vi "writeSDOU16.vi"(6 "object sub-index (0)":u8 format="%x", 7 "object index":u16 format="%x", 8 "error in (no error)":errorcluster, 9 "interface object in":refnum<k20>, 10 "inputNumber":u16, 11 "MotorController in":refnum<class "MotorController.lvclass">) -> (0 "error out":errorcluster, 1 "completion code":u32, 2 "interface object out":refnum<k20>, 3 "MotorController out":refnum<class "MotorController.lvclass">)   [LabVIEW 2017, in "MotorController.lvclass"]
uses:
  MotorController.lvclass
  MotorController.lvclass/MotorController.ctl
  <vilib>/CANopenLib/CANOPEN.llb/CANopen SDO Create.vi
  <vilib>/CANopenLib/CANOPEN.llb/CANopen SDO Write [U16].vi
  <vilib>/CANopenLib/CANOPEN.llb/CANopen SDO Close.vi
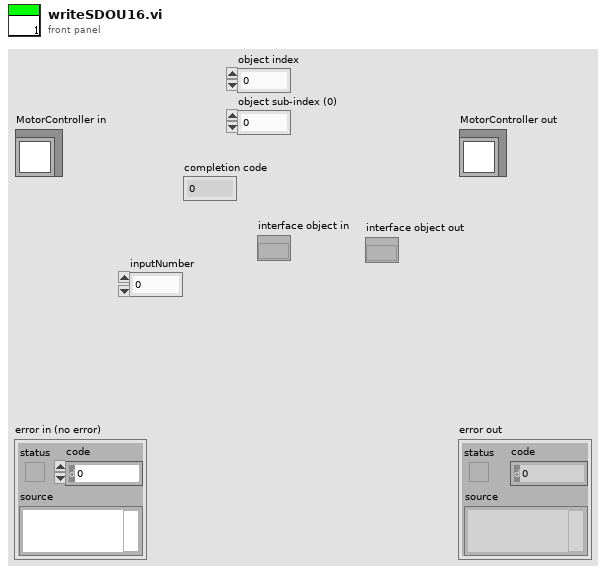
[diagram p1: front panel]
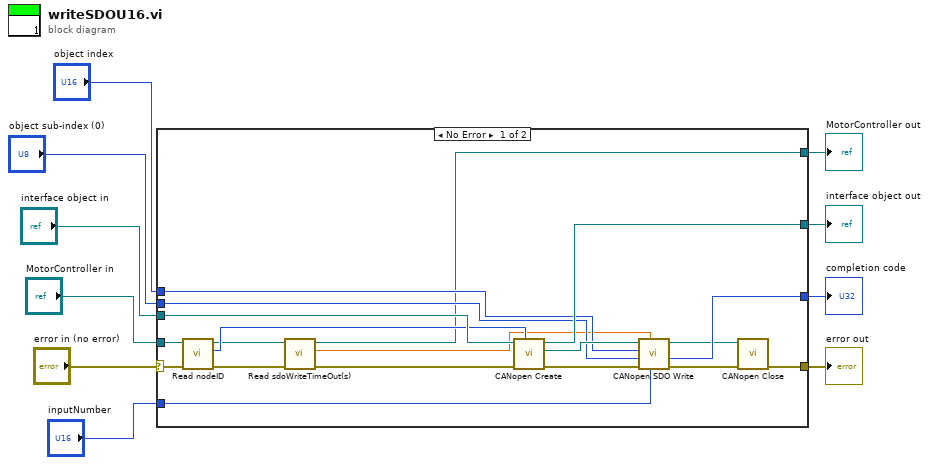
[diagram p0: block diagram]
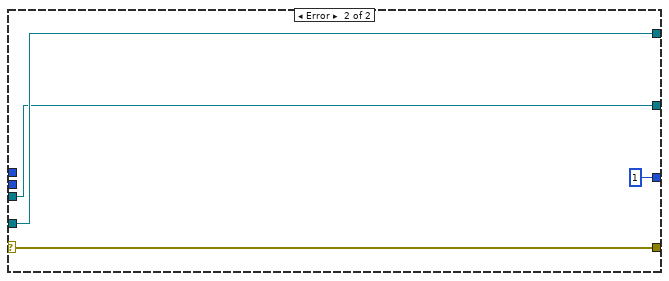
[diagram p2: hidden frame]
diagram:
  n1 = case shown="No Error" "error in (no error)" {
    selector: "error in (no error)" -> [w26 w33]
    tunnel: [w18 w33] -> w9
    tunnel: [w14 w32] -> w7
    tunnel: "MotorController in" -> [w27 w32]
    tunnel: [w29 w30] -> w6
    tunnel: "interface object in" -> [w28 w30]
    tunnel: "object index" -> [w23 _]
    tunnel: "object sub-index (0)" -> [w22 _]
    tunnel: "inputNumber" -> [w21 _]
    tunnel: [w20 u32 1 ("completion code")] -> w1
    frame No Error {
      n2 = call "Read nodeID.vi"("error in (no error)"=w26, "MotorController in"=w27) -> ("error out"=w13:errorcluster, "nodeID"=w25:u8, "MotorController out"=w15:refnum<class "MotorController.lvclass">)  [unwired: 7 in]
      n3 = call "Read sdoWriteTimeOut(s).vi"("error in (no error)"=w13, "MotorController in"=w15) -> ("error out"=w12:errorcluster, "sdoWriteTimeOut(s)"=w16:dbl, "MotorController out"=w14:refnum<class "MotorController.lvclass">)  [unwired: 7 in]
      n4 = call-poly <vilib>:"CANopen Create.vi"("node-ID"=w25, "error in (no error)"=w12, "interface object in"=w28) -> ("error out"=w11:errorcluster, "SDO object out"=w24:refnum<k20>, "interface object out"=w29:refnum<k20>)  [unwired: 6 in]
      n5 = call-poly <vilib>:"CANopen SDO Write.vi"("U16 data"=w21, "timeout (1s)"=w16, "error in (no error)"=w11, "object sub-index (0)"=w22, "object index"=w23, "SDO object in"=w24) -> ("error out"=w19:errorcluster, "completion code"=w20:u32, "SDO object out"=w17:refnum<k20>)  [unwired: 3 in]
      n6 = call-poly <vilib>:"CANopen Close.vi"("error in (no error)"=w19, "SDO object in"=w17) -> ("error out"=w18:errorcluster)  [unwired: 9 in]
    }
    frame Error {
    }
  }
  "error out" <- w9
  "MotorController out" <- w7
  "interface object out" <- w6
  "completion code" <- w1
